vi "OpenCamera.vi"(8 "error in (no error)":errorcluster, 10 "Camera ID":string, 11 "ZWO_ASI in":refnum<class "ZWO_ASI.lvclass">) -> (0 "error out":errorcluster, 3 "ZWO_ASI out":refnum<class "ZWO_ASI.lvclass">)   [LabVIEW 2023, in "ZWO_ASI.lvlib" / "ZWO_ASI.lvclass"]
uses:
  ZWO_ASI.lvclass
  ZWO_ASI.lvclass/ZWO_ASI.ctl
  <userlib>/ASICamera2_no_err/ASICamera2_no_err.lvlib
  Interfaces/InitDeinitInterface/InitDeinitComm Messages/InitDone Msg/InitDone Msg.lvclass
  <vilib>/ActorFramework/Actor/Actor.lvclass
  Applications/National Instruments/LabVIEW 2023 64-bit/vi.lib/ActorFramework/Actor/Actor.lvclass
  Users/alexandrosspiliotis/Documents/LV_DAQ_Project/ConcreteClasses/ConcreteInstrumentClasses/CameraClasses/ZWO_ASI_LV/ZWO_ASI/ZWO_ASI.lvclass
  Users/alexandrosspiliotis/Documents/LV_DAQ_Project/Interfaces/AbstractInstrumentClasses/Cameras_LV/CameraInterface/CameraInterface.lvclass
  Users/alexandrosspiliotis/Documents/LV_DAQ_Project/Interfaces/InitDeinitInterface/InitDeinit/InitDeinit.lvclass
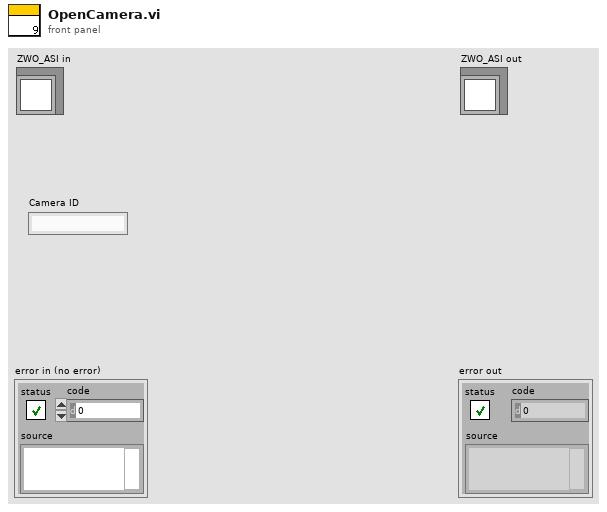
[diagram p1: front panel]
types:
  T1 = cluster{"Name[0]":i8, "Name[1]":i8, "Name[2]":i8, "Name[3]":i8, "Name[4]":i8, "Name[5]":i8, "Name[6]":i8, "Name[7]":i8, "Name[8]":i8, "Name[9]":i8, "Name[10]":i8, "Name[11]":i8, "Name[12]":i8, "Name[13]":i8, "Name[14]":i8, "Name[15]":i8, "Name[16]":i8, "Name[17]":i8, "Name[18]":i8, "Name[19]":i8, "Name[20]":i8, "Name[21]":i8, "Name[22]":i8, "Name[23]":i8, "Name[24]":i8, "Name[25]":i8, "Name[26]":i8, "Name[27]":i8, "Name[28]":i8, "Name[29]":i8, "Name[30]":i8, "Name[31]":i8, "Name[32]":i8, "Name[33]":i8, "Name[34]":i8, "Name[35]":i8, "Name[36]":i8, "Name[37]":i8, "Name[38]":i8, "Name[39]":i8, "Name[40]":i8, "Name[41]":i8, "Name[42]":i8, "Name[43]":i8, "Name[44]":i8, "Name[45]":i8, "Name[46]":i8, "Name[47]":i8, "Name[48]":i8, "Name[49]":i8, "Name[50]":i8, "Name[51]":i8, "Name[52]":i8, "Name[53]":i8, "Name[54]":i8, "Name[55]":i8, "Name[56]":i8, "Name[57]":i8, "Name[58]":i8, "Name[59]":i8, "Name[60]":i8, "Name[61]":i8, "Name[62]":i8, "Name[63]":i8, "CameraID":i32, "MaxHeight":i32, "MaxWidth":i32, "IsColorCam":u32, "BayerPattern":u32, "SupportedBins[0]":i32, "SupportedBins[1]":i32, "SupportedBins[2]":i32, "SupportedBins[3]":i32, "SupportedBins[4]":i32, "SupportedBins[5]":i32, "SupportedBins[6]":i32, "SupportedBins[7]":i32, "SupportedBins[8]":i32, "SupportedBins[9]":i32, "SupportedBins[10]":i32, "SupportedBins[11]":i32, "SupportedBins[12]":i32, "SupportedBins[13]":i32, "SupportedBins[14]":i32, "SupportedBins[15]":i32, "SupportedVideoFormat[0]":u32, "SupportedVideoFormat[1]":u32, "SupportedVideoFormat[2]":u32, "SupportedVideoFormat[3]":u32, "SupportedVideoFormat[4]":u32, "SupportedVideoFormat[5]":u32, "SupportedVideoFormat[6]":u32, "SupportedVideoFormat[7]":u32, "@dummy control@":i8, "@dummy control@":i8, "@dummy control@":i8, "@dummy control@":i8, "PixelSize":dbl, "MechanicalShutter":u32, "ST4Port":u32, "IsCoolerCam":u32, "IsUSB3Host":u32, "IsUSB3Camera":u32, "ElecPerADU":sgl, "Unused[0]":i8, "Unused[1]":i8, "Unused[2]":i8, "Unused[3]":i8, "Unused[4]":i8, "Unused[5]":i8, "Unused[6]":i8, "Unused[7]":i8, "Unused[8]":i8, "Unused[9]":i8, "Unused[10]":i8, "Unused[11]":i8, "Unused[12]":i8, "Unused[13]":i8, "Unused[14]":i8, "Unused[15]":i8, "Unused[16]":i8, "Unused[17]":i8, "Unused[18]":i8, "Unused[19]":i8, "Unused[20]":i8, "Unused[21]":i8, "Unused[22]":i8, "Unused[23]":i8}
  T2 = typedef "InstrumentData.ctl" = cluster{"Instr Error":errorcluster, "Address":cluster{"address type":enum16{"VISA", "Index"}, "Address":string, "instrument type":T3}}
  T3 = typedef "instrumentType.ctl" = enum16{"Spectrometer", "Camera", "Stepper"}
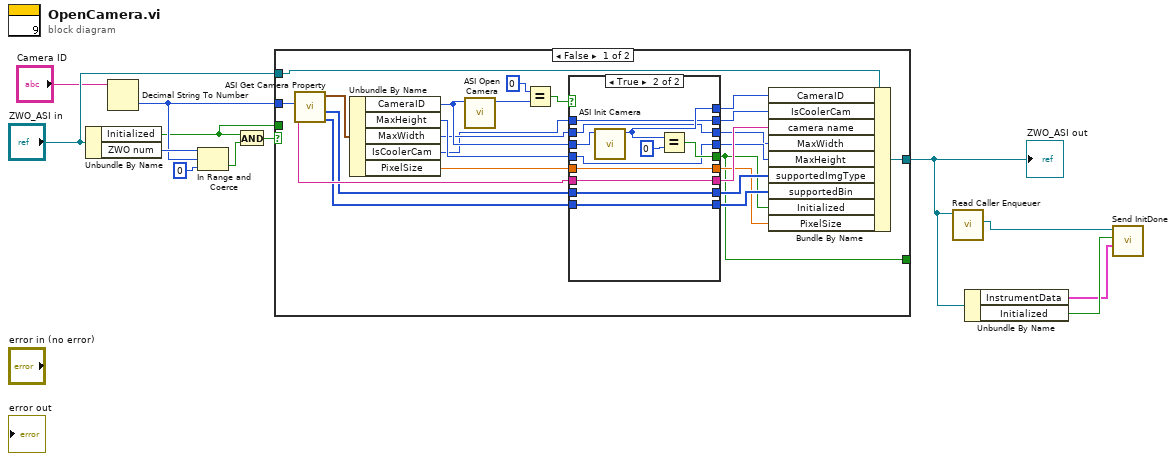
[diagram p0: block diagram]
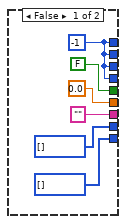
[diagram p2: hidden frame]
diagram:
  n1 = Unbundle By Name("ZWO_ASI in") -> ("Initialized"=w4:bool, "ZWO num"=w10:i32)
  n2 = Decimal String To Number(string="Camera ID") -> (number=w6:i32)  [unwired: 2 in, 1 out]
  n3 = In Range and Coerce(upper limit=w10, x=w6, lower limit=0) -> (In Range?=w8:bool)  [unwired: 1 out]
  n4 = And(x=w4, y=w8) -> (x .and. y?=w7:bool)
  n5 = case shown="False" w7 {
    tunnel: w6 -> [w31 _]
    tunnel: "ZWO_ASI in" -> [w30 w55]
    tunnel: [w29 w55] -> w3
    tunnel: [w13 w54] -> _
    tunnel: w4 -> [_ w54]
    frame False {
      n6 = call <userlib>:"ASI Get Camera Property.vi"("iCameraIndex"=w31) -> ("supportedBin"=w22:i8[], "supportedImgType"=w21:i8[], "pASICameraInfo out"=w34:T1, "cameraName"=w26:string)  [unwired: 6 in, 1 out]
      n7 = Unbundle By Name(w34) -> ("CameraID"=w32:i32, "MaxHeight"=w24:i32, "MaxWidth"=w17:i32, "IsCoolerCam"=w16:u32, "PixelSize"=w15:dbl)
      n8 = call <userlib>:"ASI Open Camera.vi"("iCameraID"=w32) -> ("function return"=w36:i32)  [unwired: 10 in]
      n9 = Equal?(x=0, y=w36) -> (x = y?=w33:bool)
      n10 = case shown="True" w33 {
        tunnel: [FALSE w52] -> w13
        tunnel: w32 -> [_ w51]
        tunnel: [w41 w50] -> w28
        tunnel: [w41 w44] -> w27
        tunnel: w26 -> [_ w49]
        tunnel: ["" ("cameraName") w49] -> w25
        tunnel: w24 -> [_ w46]
        tunnel: [i8[] [] ("supportedBin") w48] -> w23
        tunnel: w22 -> [_ w48]
        tunnel: w21 -> [_ w47]
        tunnel: [i8[] [] ("supportedImgType") w47] -> w20
        tunnel: [w41 w46] -> w19
        tunnel: [w41 w45] -> w18
        tunnel: w17 -> [_ w45]
        tunnel: w16 -> [_ w44]
        tunnel: w15 -> [_ w43]
        tunnel: [0.0 ("PixelSize") w43] -> w14
        frame False {
          w41 = -1 ("function return")
        }
        frame True {
          n11 = call <userlib>:"ASI Init Camera.vi"("iCameraID"=w51) -> ("function return"=w50:i32)  [unwired: 10 in]
          n12 = Equal?(x=w50, y=0 ("x")) -> (x = y?=w52:bool)
        }
      }
      n13 = Bundle By Name(cluster=w30, "CameraID"=w28, "IsCoolerCam"=w27, "camera name"=w25, "MaxWidth"=w18, "MaxHeight"=w19, "supportedImgType"=w20, "supportedBin"=w23, "Initialized"=w13, "PixelSize"=w14) -> (w29:refnum<class "ZWO_ASI.lvclass">)
    }
    frame True {
    }
  }
  "ZWO_ASI out" <- w3
  n14 = call <vilib>:"Read Caller Enqueuer.vi"("Actor"=w3) -> ("Caller Enqueuer"=w5:refnum<class "Message Enqueuer.lvclass">)  [unwired: 10 in]
  n15 = Unbundle By Name(w3) -> ("InstrumentData"=w1:T2, "Initialized"=w2:bool)
  n16 = call "Send InitDone.vi"("InstrumentData"=w1, "Initialized"=w2, "Message Enqueuer"=w5) -> ()  [unwired: 7 in, 2 out]
